vi "GenerateFakeSignal.vi"(9 "SecondaryDataVIRef":refnum<vi>, 10 "Array":sgl[](array[numeric])) -> (2 "simulated signal":sgl[](array[numeric]))   [LabVIEW 2014, in "GenericDAQ.lvlib"]
uses:
  <instrlib>/GenericDAQ/GenericDAQ.lvlib
  <vilib>/gmath/SpecialFunctions.llb/Error Function.vi
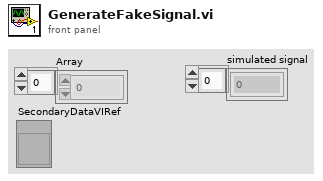
[diagram p1: front panel]
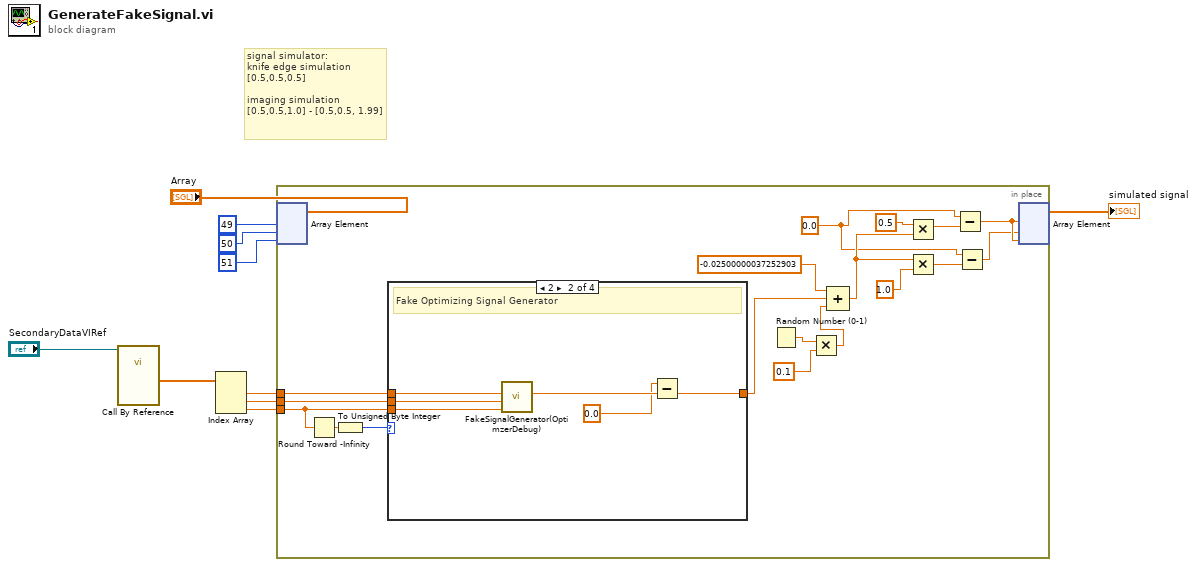
[diagram p0: block diagram]
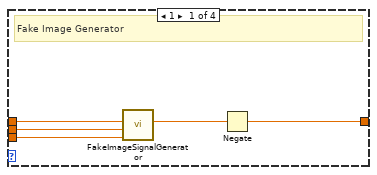
[diagram p2: hidden frame]
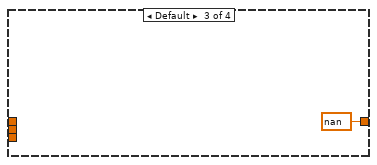
[diagram p3: hidden frame]
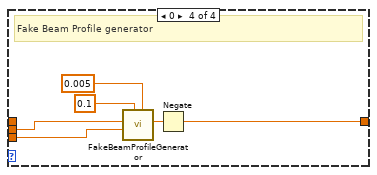
[diagram p4: hidden frame]
diagram:
  # "signal simulator:\nknife edge simulation\n[0.5,0.5,0.5]\n\nimaging simulation\n[0.5,0.5,1.0] - [0.5,0.5, 1.99]"
  n1 = call-by-ref "?"(reference="SecondaryDataVIRef") -> ("SecondaryData"=w7:dbl[])  [unwired: 12 in, 2 out]
  n2 = Index Array(array=w7) -> (element #1=w6:dbl, element #2=w5:dbl, element #3=w4:dbl)  [unwired: 3 in]
  n3 = in-place {
    in-place-border: w6 -> [w16]
    in-place-border: w5 -> [w15]
    in-place-border: w4 -> [w12]
    w14 = sgl 0.0
    n4 = in-place-array #1("Array", 49, 50, 51) -> ()  [unwired: 3 out]
    n5 = Round Toward -Infinity(1:w12) -> (0:w13:dbl)
    n6 = To Unsigned Byte Integer(number=w13) -> (unsigned 8bit integer=w11:u8)
    n7 = case shown="2" w11 {
      tunnel: [w29 w35 nan w46] -> w25
      tunnel: w16 -> [w32 w38 _ _]
      tunnel: w15 -> [w31 w37 _ w41]
      tunnel: w12 -> [w30 w36 _ w42]
      frame 1 {
        # "Fake Image Generator"
        n8 = call <instrlib>:"FakeImageSignalGenerator.vi"("Z"=w30, "Y"=w31, "X"=w32) -> ("E"=w33:dbl)  [unwired: 8 in]
        n9 = Negate(x=w33) -> (-x=w29:dbl)
      }
      frame 2 {
        # "Fake Optimizing Signal Generator"
        n10 = call <instrlib>:"FakeSignalGenerator(OptimzerDebug).vi"("Z"=w36, "Y"=w37, "X"=w38) -> ("E"=w39:dbl)  [unwired: 8 in]
        n11 = Subtract(x=0.0 ("E"), y=w39) -> (x-y=w35:dbl)
      }
      frame Default {
      }
      frame 0 {
        # "Fake Beam Profile generator"
        n12 = call <instrlib>:"FakeBeamProfileGenerator.vi"("w_0"=0.005, "Z_0"=0.1, "Z"=w42, "Y"=w41) -> ("E"=w45:dbl)  [unwired: 7 in]
        n13 = Negate(x=w45) -> (-x=w46:dbl)
      }
    }
    n14 = Random Number (0-1)() -> (number: 0 to 1=w26:dbl)
    n15 = Multiply(x=w26, y=0.1) -> (x*y=w28:dbl)
    n16 = Compound Arithmetic op=ADD(-0.02500000037252903 ("value"), w25, w28) -> (w24:dbl)
    n17 = Multiply(x=0.5, y=w24) -> (x*y=w21:dbl)
    n18 = Multiply(x=w24, y=1.0 ("x*y")) -> (x*y=w18:dbl)
    n19 = Subtract(x=w14, y=w21) -> (x-y=w20:dbl)
    n20 = Subtract(x=w14, y=w18) -> (x-y=w19:dbl)
    n21 = in-place-array #1(w20, w19, w20) -> (→"simulated signal":sgl[])  [unwired: 3 out]
  }
